vi "Add Local Variable (Double Array).vi"(8 "error in (no error)":errorcluster, 9 "Array":dbl[](array[numeric]), 10 "Identifier":string, 11 "Sequence Ref in":refnum<k24>) -> (0 "error out":errorcluster, 3 "Sequence Ref out":refnum<k24>)   [LabVIEW 2015, in "Single Station Execution.lvlib"]
uses:
  Single Station Execution.lvlib
  NationalInstruments.VeriStand.RealTimeSequenceDefinitionApi
  NationalInstruments.VeriStand.DataTypes
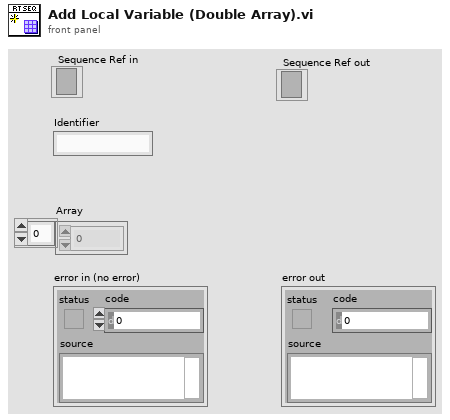
[diagram p1: front panel]
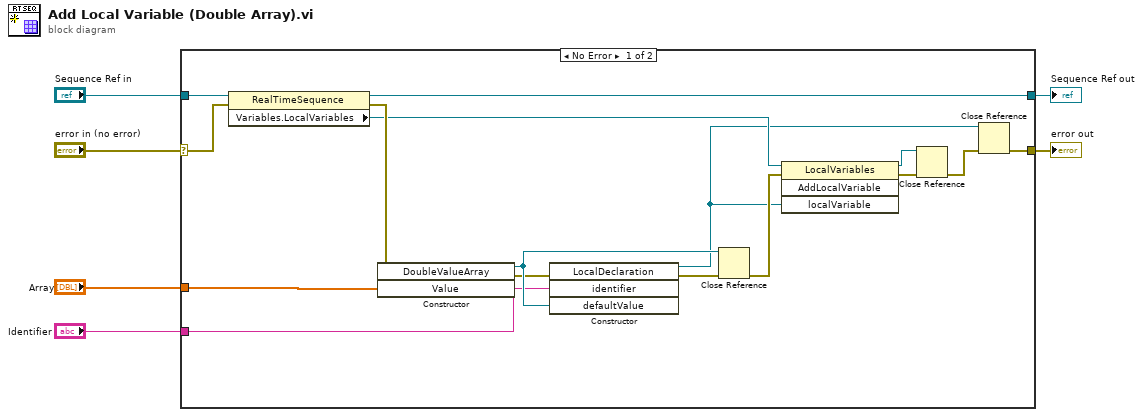
[diagram p0: block diagram]
diagram:
  n1 = case shown="No Error" "error in (no error)" {
    selector: "error in (no error)" -> [w7 w23]
    tunnel: "Array" -> [w19 _]
    tunnel: "Identifier" -> [w16 _]
    tunnel: "Sequence Ref in" -> [w15 w24]
    tunnel: [w14 w24] -> w3
    tunnel: [w10 w23] -> w2
    frame No Error {
      n2 = property class="RealTimeSequence"(reference=w15, error in=w7) -> (reference out=w14:refnum<k24>, error out=w18:errorcluster, "Variables.LocalVariables"=w17:refnum<k24>)
      n3 = constructor class="DoubleValueArray"(error in=w18, "Value"=w19) -> (reference out=w21:refnum<k24>, error out=w20:errorcluster)  [unwired: 2 in, 2 out]
      n4 = constructor class="LocalDeclaration"(error in=w20, "identifier"=w16, "defaultValue"=w21) -> (reference out=w8:refnum<k24>, error out=w13:errorcluster)  [unwired: 2 in, 3 out]
      n5 = Close Reference(reference=w21, error in (no error)=w13) -> (error out=w22:errorcluster)
      n6 = invoke class="LocalVariables" method="AddLocalVariable"(reference=w17, error in=w22, "localVariable"=w8) -> (reference out=w9:refnum<k24>, error out=w12:errorcluster)  [unwired: 1 in, 2 out]
      n7 = Close Reference(reference=w9, error in (no error)=w12) -> (error out=w11:errorcluster)
      n8 = Close Reference(reference=w8, error in (no error)=w11) -> (error out=w10:errorcluster)
    }
    frame Error {
    }
  }
  "Sequence Ref out" <- w3
  "error out" <- w2
